vi "Create Map from Messages to Value Indexes.vi"(8 "error in":errorcluster, 9 "hardware handles":T3, 10 "1553 channel handles":T4[](array[typedef]) {"terminal status channels" format="%.0x"; "error count channel refs"."wrong sync" format="%.0x"; "error count channel refs"."word" format="%.0x"; "error count channel refs"."unconfigured frames" format="%.0x"; "error count channel refs"."parity" format="%.0x"; "error count channel refs"."monitor" format="%.0x"; "error count channel refs"."Manchester" format="%.0x"; "error count channel refs"."improper number of words" format="%.0x"; "error count channel refs"."general protocol" format="%.0x"; "messages"."Rx status handles" format="%.0x"; "messages"."Tx status handles" format="%.0x"; "messages"."timestamps" format="%.0x"; "messages"."parameters"."RxBC channel handle" format="%.0x"; "messages"."parameters"."RxRT channel handle" format="%.0x"; "messages"."parameters"."Tx channel handle" format="%.0x"}, 11 "1553 channels":T9[](array[typedef])) -> (0 "error out":errorcluster, 1 "Rx read info":T1[](array[typedef]), 2 "status lookup data":T2[](array[typedef]) {"terminal address" format="%.0x"; "remote terminal handle" format="%.0x"}, 3 "map from messages to value indexes":T15)   [LabVIEW 2020, in "Ballard MIL-STD-1553 Engine.lvlib" / "Custom Device.lvlib"]
uses:
  Custom Device.lvlib
  Shared/Map of Messages to Value Indexes.ctl
  Shared/Message Map Key.ctl
  Implementation/Rx Execution Unit/Message Map Value.ctl
  Shared/Message Definition.ctl
  Shared/Message Type.ctl
  Shared/Terminal Endpoint.ctl
  Shared/Address.ctl
  Shared/Parameter Definition.ctl
  Shared/1553 Channel.ctl
  Implementation/Execution Unit/1553 Channel Handles.ctl
  Implementation/Execution Unit/Message Handles.ctl
  Implementation/Execution Unit/Parameter Handles.ctl
  <vilib>/NI VeriStand/Custom Device API/Custom Device Item Ref.ctl
  Shared/Error Count Channel Refs.ctl
  Hardware Handles.ctl
  Implementation/Rx Execution Unit/Status Terminal Lookup Data.ctl
  Shared/Rx Read Info.ctl
  Implementation/Rx Execution Unit/Rx Execution Unit.lvclass
  <vilib>/NI VeriStand/Custom Device API/Custom Device API.lvlib
  Implementation/Execution Unit/Execution Unit.lvclass
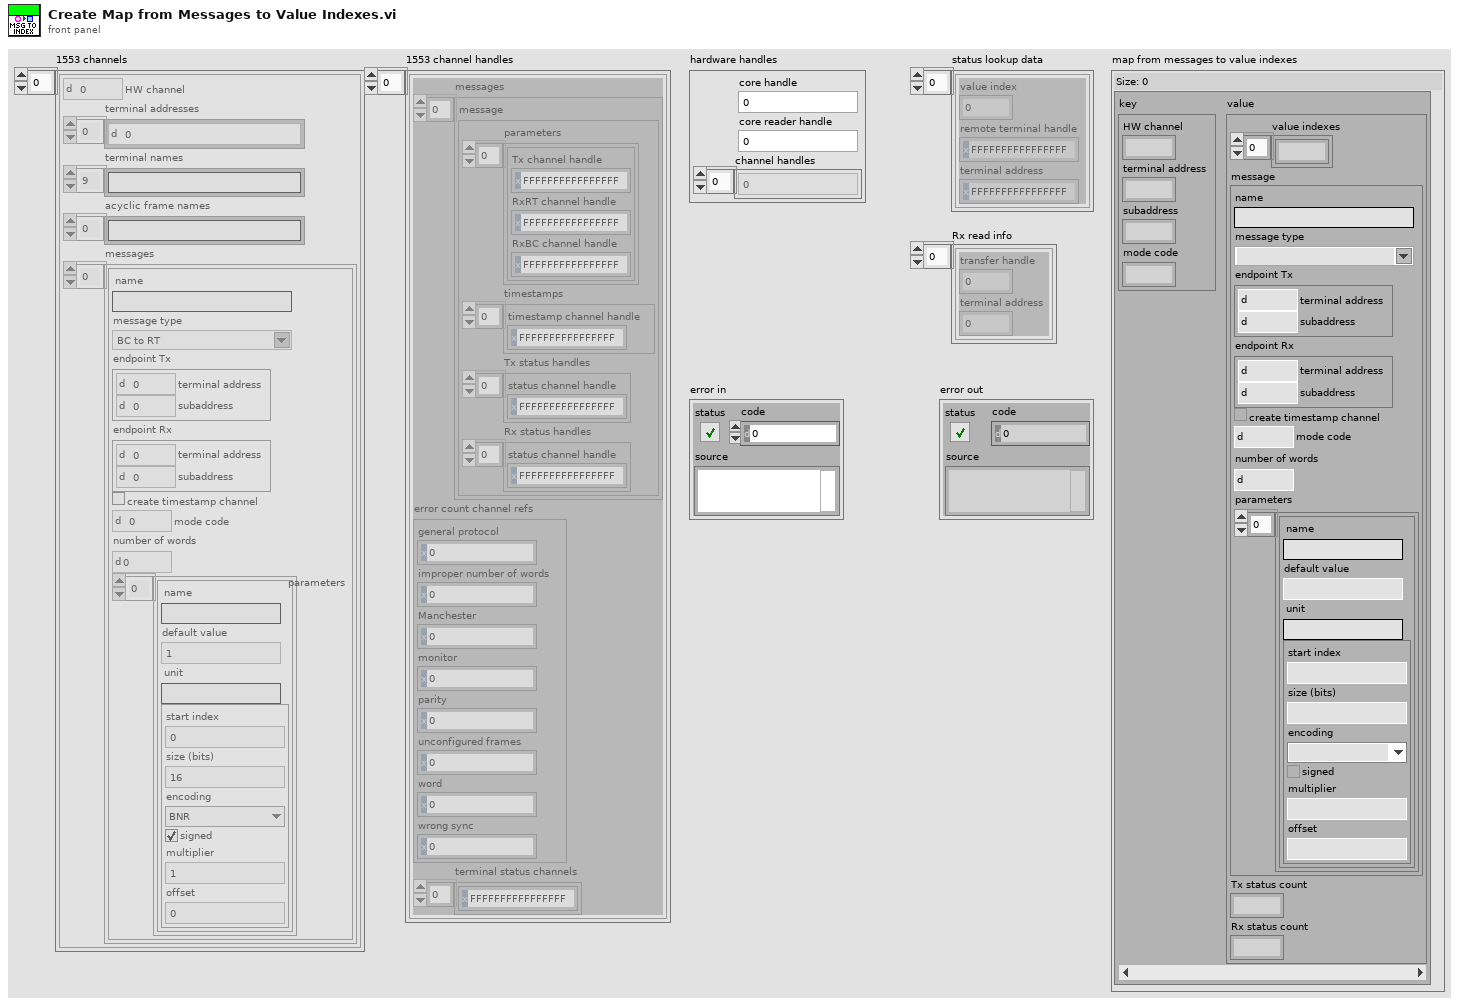
[diagram p1: front panel]
types:
  T1 = typedef "Rx Read Info.ctl" = cluster{"transfer handle":u64, "terminal address":u16}
  T2 = typedef "Ballard MIL-STD-1553 Engine.lvlib/Implementation.lvlib/Rx Execution Unit.lvclass/Status Terminal Lookup Data.ctl" = cluster{"value index":i32, "remote terminal handle":u64, "terminal address":u64}
  T3 = typedef "Ballard MIL-STD-1553 Engine.lvlib/Custom Device.lvlib/Hardware Handles.ctl" = cluster{"core handle":u64, "core reader handle":u64, "channel handles":u64[]}
  T4 = typedef "Ballard MIL-STD-1553 Engine.lvlib/Implementation.lvlib/Execution Unit.lvclass/1553 Channel Handles.ctl" = cluster{"messages":T5[], "error count channel refs":T8, "terminal status channels":T7[]}
  T5 = typedef "Ballard MIL-STD-1553 Engine.lvlib/Implementation.lvlib/Execution Unit.lvclass/Message Handles.ctl" = cluster{"parameters":T6[], "timestamps":T7[], "Tx status handles":T7[], "Rx status handles":T7[]}
  T6 = typedef "Ballard MIL-STD-1553 Engine.lvlib/Implementation.lvlib/Execution Unit.lvclass/Parameter Handles.ctl" = cluster{"Tx channel handle":T7, "RxRT channel handle":T7, "RxBC channel handle":T7}
  T7 = typedef "Custom Device API.lvlib/Custom Device Item Ref.ctl" = u64
  T8 = typedef "Error Count Channel Refs.ctl" = cluster{"general protocol":T7, "improper number of words":T7, "Manchester":T7, "monitor":T7, "parity":T7, "unconfigured frames":T7, "word":T7, "wrong sync":T7}
  T9 = typedef "1553 Channel.ctl" = cluster{"HW channel":u16, "terminal addresses":T10[], "terminal names":string[], "acyclic frame names":string[], "messages":T11[]}
  T10 = typedef "Address.ctl" = u16
  T11 = typedef "Message Definition.ctl" = cluster{"name":string, "message type":T12, "endpoint Tx":T13, "endpoint Rx":T13, "create timestamp channel":bool, "mode code":u16, "number of words":u16, "parameters":cluster{"name":string, "default value":dbl, "unit":string, "parameter definition":T14}[]}
  T12 = typedef "Message Type.ctl" = string
  T13 = typedef "Terminal Endpoint.ctl" = cluster{"terminal address":T10, "subaddress":T10}
  T14 = typedef "Parameter Definition.ctl" = cluster{"start index":i32, "size (bits)":i32, "encoding":enum16{"BNR", "BCD", "Discrete"}, "signed":bool, "multiplier":dbl, "offset":dbl}
  T15 = typedef "Map of Messages to Value Indexes.ctl" = map{T16, T17}
  T16 = typedef "Message Map Key.ctl" = cluster{"HW channel":u16, "terminal address":u16, "subaddress":u16, "mode code":u16}
  T17 = typedef "Ballard MIL-STD-1553 Engine.lvlib/Implementation.lvlib/Rx Execution Unit.lvclass/Message Map Value.ctl" = cluster{"value indexes":i32[], "message":T11, "Tx status count":i32, "Rx status count":i32}
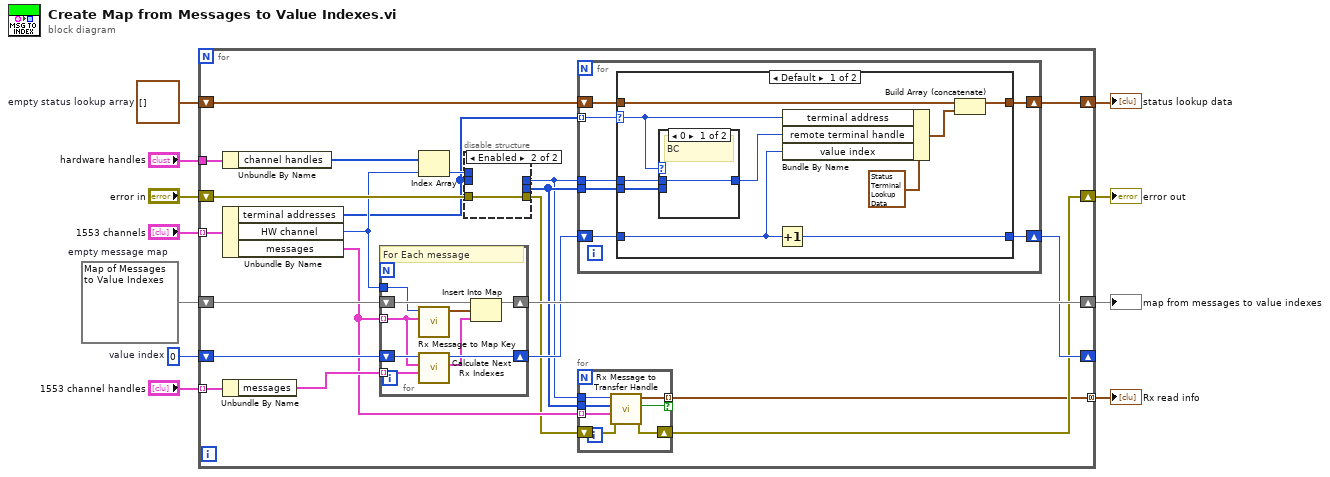
[diagram p0: block diagram]
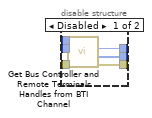
[diagram p2: hidden frame]
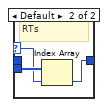
[diagram p3: hidden frame]
diagram:
  w3 = T2[] []  # empty status lookup array
  w9 = 0  # value index
  w11 = T15 {}  # empty message map
  n1 = for {
    tunnel: "1553 channels" -> [w29] mode=indexing
    shift-right: [w31] -> w7
    shift-left: w11 -> [w33]
    shift-right: [w22] -> _
    shift-left: w9 -> [w32]
    tunnel: "1553 channel handles" -> [w25] mode=indexing
    tunnel: "hardware handles" -> [w27]
    shift-right: [w13] -> w5
    shift-left: "error in" -> [w21]
    shift-right: [w24] -> w2
    shift-left: w3 -> [w28]
    tunnel: [w12] -> w1 mode=concatenating
    n2 = Unbundle By Name(w27) -> ("channel handles"=w26:u64[])
    n3 = Unbundle By Name(w29) -> ("terminal addresses"=w18:T10[], "HW channel"=w19:u16, "messages"=w17:T11[])
    n4 = Unbundle By Name(w25) -> ("messages"=w30:T5[])
    n5 = for {
      tunnel: w19 -> [w54]
      tunnel: w17 -> [w50] mode=indexing
      shift-right: [w56] -> w31
      shift-left: w33 -> [w55]
      shift-right: [w53] -> w23
      shift-left: w32 -> [w52]
      tunnel: w30 -> [w48] mode=indexing
      # "For Each message"
      n6 = call "Rx Message to Map Key.vi"("message"=w50, "HW channel"=w54) -> ("message map key"=w51:T16)  [unwired: 9 in]
      n7 = call "Calculate Next Rx Indexes.vi"("message handles"=w48, "message"=w50, "index"=w52) -> ("message map value"=w49:T17, "next index"=w53:i32)  [unwired: 7 in]
      n8 = Insert Into Map(map in=w55, key=w51, value=w49) -> (map out=w56:T15)  [unwired: 2 out]
    }
    n9 = Index Array(array=w26, index=w19) -> (element=w20:u64)
    n10 = disable-structure shown="Enabled" {
      disable-tunnel: w21 -> [w39 w40]
      disable-tunnel: w20 -> [w38 _]
      disable-tunnel: w18 -> [w37 _]
      disable-tunnel: [w36 _] -> w16
      disable-tunnel: [w35 _] -> w15
      disable-tunnel: [w34 w40] -> w14
      frame Disabled {
        n11 = call "Get Bus Controller and Remote Terminals Handles from BTI Channel.vi"("error in"=w39, "terminal addresses"=w37, "channel handle in"=w38) -> ("error out"=w34:errorcluster, "remote terminal handles out"=w36:u64[], "bus controller handle out"=w35:u64)  [unwired: 5 in, 1 out]
      }
      frame Enabled {
      }
    }
    n12 = for {
      tunnel: w18 -> [w57] mode=indexing
      shift-right: [w63] -> w24
      shift-left: w28 -> [w62]
      tunnel: w16 -> [w61]
      tunnel: w15 -> [w60]
      shift-right: [w58] -> w22
      shift-left: w23 -> [w59]
      n13 = case shown="Default" w57 {
        selector: w57 -> [w65 _]
        tunnel: [w67 w79] -> w63
        tunnel: w62 -> [w68 w79]
        tunnel: w61 -> [w73 _]
        tunnel: w60 -> [w72 _]
        tunnel: w59 -> [w64 w78]
        tunnel: [w69 w78] -> w58
        frame Default {
          n14 = case shown="0" w65 {
            selector: w65 -> [_ w76]
            tunnel: w73 -> [_ w77]
            tunnel: w72 -> [w74 _]
            tunnel: [w74 w75] -> w70
            frame 0 {
              # "BC"
            }
            frame Default {
              # "RTs"
              n15 = Index Array(array=w77, index=w76) -> (element=w75:u64)
            }
          }
          n16 = Increment(x=w64) -> (x+1=w69:i32)
          n17 = Bundle By Name(cluster=T2 {"value index"=0, "remote terminal handle"=18446744073709551615, "terminal address"=18446744073709551615} ("value"), "terminal address"=w65, "remote terminal handle"=w70, "value index"=w64) -> (w66:T2)
          n18 = Build Array (concatenate)(w68, w66) -> (w67:T2[])
        }
        frame 31 {
        }
      }
    }
    n19 = for {
      tunnel: w17 -> [w45] mode=indexing
      tunnel: w16 -> [w46]
      tunnel: w15 -> [w47]
      shift-right: [w43] -> w13
      shift-left: w14 -> [w44]
      tunnel: [w42] -> w12 mode=indexing if=w41
      n20 = call "Rx Message to Transfer Handle.vi"("error in"=w44, "message"=w45, "remote terminal handles"=w46, "bus controller handle"=w47) -> ("error out"=w43:errorcluster, "valid?"=w41:bool, "Rx read info"=w42:T1)  [unwired: 5 in]
    }
  }
  "map from messages to value indexes" <- w7
  "error out" <- w5
  "status lookup data" <- w2
  "Rx read info" <- w1
